vi "Passed.vi"(1 "TestResult In":refnum<class "TestResult.lvclass">) -> (0 "Passed":refnum<class "Test.lvclass">[](array[class]))   [LabVIEW 2019, in "TestResult.lvclass"]
doc: "Returns the list of passed tests."
uses:
  TestResult.lvclass
  TestResult.lvclass/TestResult.ctl
  Test/Test.lvclass
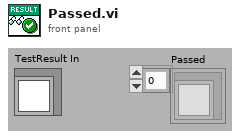
[diagram p1: front panel]
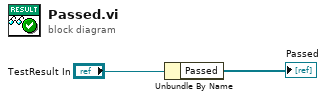
[diagram p0: block diagram]
diagram:
  n1 = Unbundle By Name("TestResult In") -> ("Passed"=→"Passed":refnum<class "Test.lvclass">[])
